vi "Actor Create.vi"(9 "Nest Alias":string, 10 "Nest Actor":refnum<class "Actor.lvclass">, 11 "Actor Create Msg Strategy in":refnum<class "Actor Create Msg Strategy.lvclass">) -> (0 "error out":errorcluster, 3 "Actor Create Msg Strategy out":refnum<class "Actor Create Msg Strategy.lvclass">)   [LabVIEW 2021, in "Actor Create.lvlib" / "Actor Create Msg Strategy.lvclass"]
uses:
  Actor Create Msg Strategy.lvclass
  LVCAM/Actor/Actor.lvclass
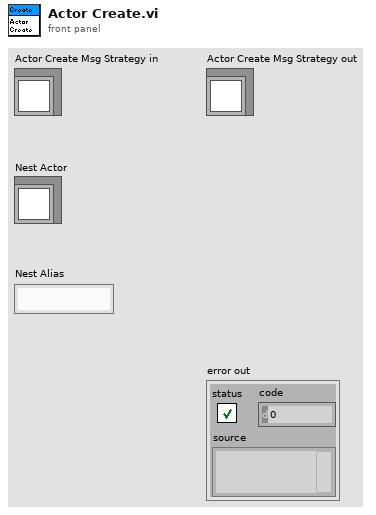
[diagram p1: front panel]
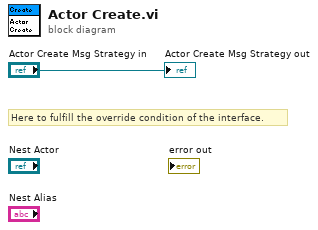
[diagram p0: block diagram]
diagram:
  # "Here to fulfill the override condition of the interface."
  "Actor Create Msg Strategy out" <- "Actor Create Msg Strategy in"
